vi "Get Endpoints from Topology.vi"(8 "error in":errorcluster, 11 "topology":string) -> (0 "error out":errorcluster, 3 "endpoints":string[](array[string]))   [LabVIEW 2017, in "NI-SWITCH Scripting.lvlib"]
uses:
  NI-SWITCH Scripting.lvlib
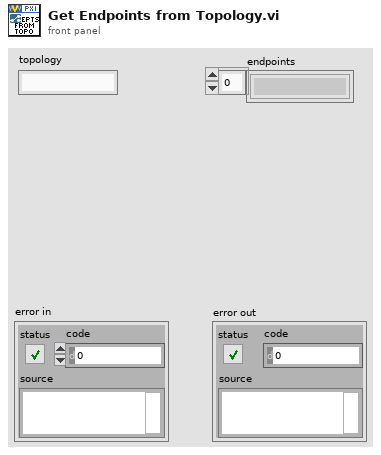
[diagram p1: front panel]
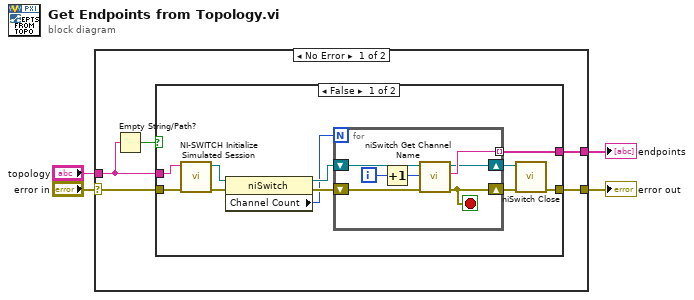
[diagram p0: block diagram]
diagram:
  n1 = case shown="No Error" "error in" {
    selector: "error in" -> [w9 w29]
    tunnel: "topology" -> [w7 _]
    tunnel: [w8 w29] -> w2
    tunnel: [w5 _] -> w1
    frame No Error {
      n2 = Empty String/Path?(string/path=w7) -> (empty?=w6:bool)
      n3 = case shown="False" w6 {
        tunnel: w9 -> [w20 w28]
        tunnel: [w12 w28] -> w8
        tunnel: w7 -> [w19 _]
        tunnel: [w10 _] -> w5
        frame False {
          n4 = call "NI-SWITCH Initialize Simulated Session.vi"("error in (no error)"=w20, "topology"=w19) -> ("error out"=w18:errorcluster, "NI-SWITCH session"=w17:refnum<k15>)  [unwired: 8 in]
          n5 = property class="niSwitch"(reference=w17, error in=w18) -> (reference out=w15:refnum<k15>, error out=w16:errorcluster, "Channel Count"=w14:i32)
          n6 = for {
            N: w14 -> [_]
            tunnel: [w25] -> w10 mode=indexing
            shift-right: [w21] -> w13
            shift-left: w16 -> [w26]
            shift-right: [w22] -> w11
            shift-left: w15 -> [w27]
            i -> [w24]
            stop <- w21 stop-if-true
            n7 = Increment(x=w24) -> (x+1=w23:i32)
            n8 = call <instrlib>:"niSwitch Get Channel Name.vi"("error in (no error)"=w26, "index (1)"=w23, "instrument handle"=w27) -> ("error out"=w21:errorcluster, "channel string"=w25:string, "instrument handle out"=w22:refnum<k15>)  [unwired: 6 in]
          }
          n9 = call <instrlib>:"niSwitch Close.vi"("error in (no error)"=w13, "instrument handle"=w11) -> ("error out"=w12:errorcluster)  [unwired: 9 in]
        }
        frame True {
        }
      }
    }
    frame Error {
    }
  }
  "error out" <- w2
  "endpoints" <- w1
